vi "OEE_SCREEN_2_map_worst_pace_record_to_cluster.vi"(11 "pace_record":i32[](array[numeric])) -> (2 "pace":string, 3 "station":string)   [LabVIEW 2019]
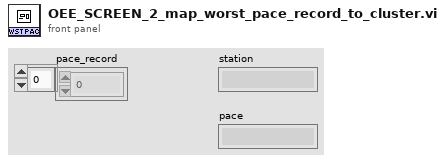
[diagram p1: front panel]
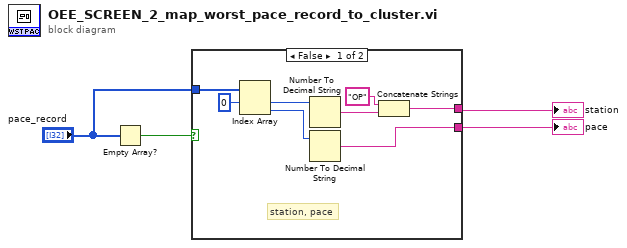
[diagram p0: block diagram]
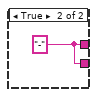
[diagram p2: hidden frame]
diagram:
  n1 = Empty Array?(array="pace_record") -> (empty?=w2:bool)
  n2 = case shown="False" w2 {
    tunnel: "pace_record" -> [w12 _]
    tunnel: [w6 w13] -> w3
    tunnel: [w5 w13] -> w4
    frame False {
      # "station, pace"
      n3 = Index Array(array=w12, index #1=0 ("index")) -> (element #1=w10:i32, element #2=w9:i32)  [unwired: 1 in]
      n4 = Number To Decimal String(number=w10) -> (decimal integer string=w8:string)  [unwired: 1 in]
      n5 = Number To Decimal String(number=w9) -> (decimal integer string=w5:string)  [unwired: 1 in]
      n6 = Concatenate Strings("OP" ("string"), w8) -> (w6:string)
    }
    frame True {
      w13 = "-"
    }
  }
  "pace" <- w4
  "station" <- w3
